vi "PID Control.vi"(7 "Upwards f":dbl, 8 "Setpoint":dbl format="%.2f", 9 "PID Down":T1={"proportional gain (Kc)"=1.0, "integral time (Ti, min)"=0.01, "derivative time (Td, min)"=0.0} {"derivative time (Td, min)" format="%.3f"; "integral time (Ti, min)" format="%.3f"; "proportional gain (Kc)" format="%.3f"}, 10 "PID Up":T1={"proportional gain (Kc)"=1.0, "integral time (Ti, min)"=0.01, "derivative time (Td, min)"=0.0} {"derivative time (Td, min)" format="%.3f"; "integral time (Ti, min)" format="%.3f"; "proportional gain (Kc)" format="%.3f"}, 11 "Position":dbl format="%.2f") -> (2 "x+y":dbl)   [LabVIEW 2018]
uses:
  <vilib>/addons/control/pid/pid.llb/PID (DBL).vi
  <vilib>/addons/control/pid/NI_PID_pid.lvlib
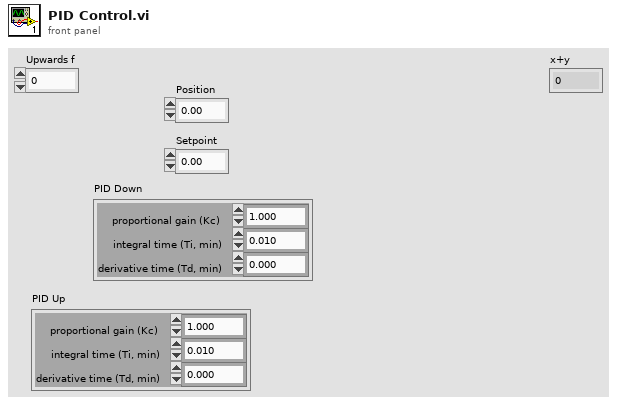
[diagram p1: front panel]
types:
  T1 = cluster{"proportional gain (Kc)":dbl, "integral time (Ti, min)":dbl, "derivative time (Td, min)":dbl}
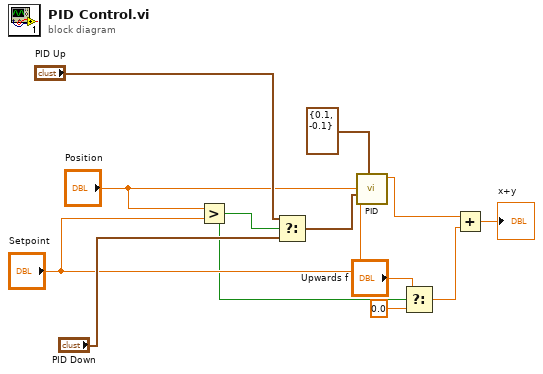
[diagram p0: block diagram]
diagram:
  n1 = Greater?(x="Position", y="Setpoint") -> (0:w6:bool)
  n2 = Select(t="PID Up", s=w6, f="PID Down") -> (s? t:f=w9:T1)
  n3 = call-poly <vilib>:"PID.vi"("output range"=cluster{"output high":dbl, "output low":dbl} {"output high"=0.1, "output low"=-0.1}, "PID gains"=w9, "process variable"="Position", "setpoint"="Setpoint") -> ("output"=w3:dbl)  [unwired: 6 in, 1 out]
  n4 = Select(t="Upwards f", s=w6, f=0.0) -> (s? t:f=w2:dbl)
  n5 = Add(x=w3, y=w2) -> (x+y=→"x+y":dbl)
